vi "T flipflop.vi"() -> ()   [LabVIEW 2020]
panel:
  in  "CLOCK":bool
  out "Q'":bool
  out "Q":bool
  in  "T":bool
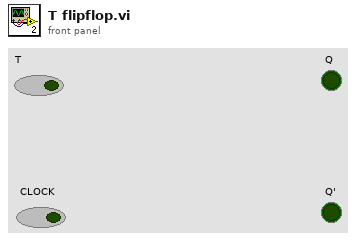
[diagram p1: front panel]
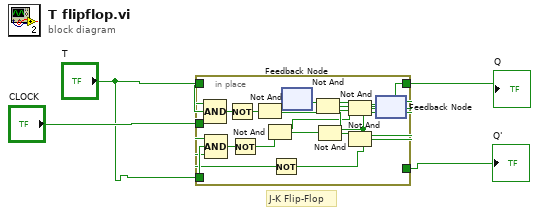
[diagram p0: block diagram]
diagram:
  # "J-K Flip-Flop"
  n1 = in-place {
    in-place-border: "T" -> [w15]
    in-place-border: "T" -> [w14]
    in-place-border: "CLOCK" -> [w12]
    in-place-border: [w10] -> w3
    in-place-border: [w9] -> w2
    n2 = Not(x=w12) -> (.not. x?=w13:bool)
    n3 = feedback #1() -> (w18:bool)  [unwired: 1 in]
    n4 = Not And(1:w13, 2:w18) -> (0:w17:bool)
    n5 = feedback #2() -> (w9:bool)  [unwired: 1 in]
    n6 = Compound Arithmetic op=AND(w12, w14, w9) -> (w6:bool)
    n7 = Not(x=w6) -> (.not. x?=w5:bool)
    n8 = Not And(1:w5, 2:w18) -> (0:w20:bool)
    n9 = Not And(1:w20, 2:w13) -> (0:w16:bool)
    n10 = Not And(1:w16, 2:w9) -> (0:w10:bool)
    n11 = Compound Arithmetic op=AND(w10, w15, w12) -> (w8:bool)
    n12 = Not(x=w8) -> (.not. x?=w7:bool)
    n13 = Not And(1:w20, 2:w7) -> (0:w19:bool)
    n14 = feedback-in #1(w19) -> ()
    n15 = Not And(1:w10, 2:w17) -> (0:w11:bool)
    n16 = feedback-in #2(w11) -> ()
  }
  "Q" <- w2
  "Q'" <- w3
